vi "laser-shutter-control-subvi.vi"(7 "Camera Shutter":bool, 8 "error in":errorcluster, 9 "VISA resource name out":refnum<visa-resource-name>, 10 "Wheel Speed":u8, 11 "Laser Shutter":T1) -> (0 "error out":errorcluster, 1 "Status":bool, 3 "Current Filterwheel":string)   [LabVIEW 2014]
uses:
  ctts/laser shutters.ctl
  Global Shutter Variables - SubVI.vi
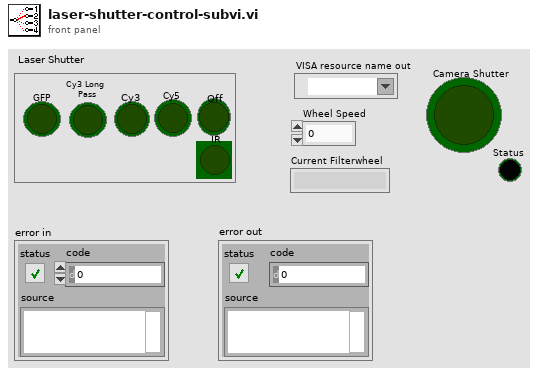
[diagram p1: front panel]
types:
  T1 = typedef "laser shutters.ctl" = enum32{"No Selection", "GFP", "Cy3 Long \nPass", "Cy3", "Cy5", "Off", "IR"}
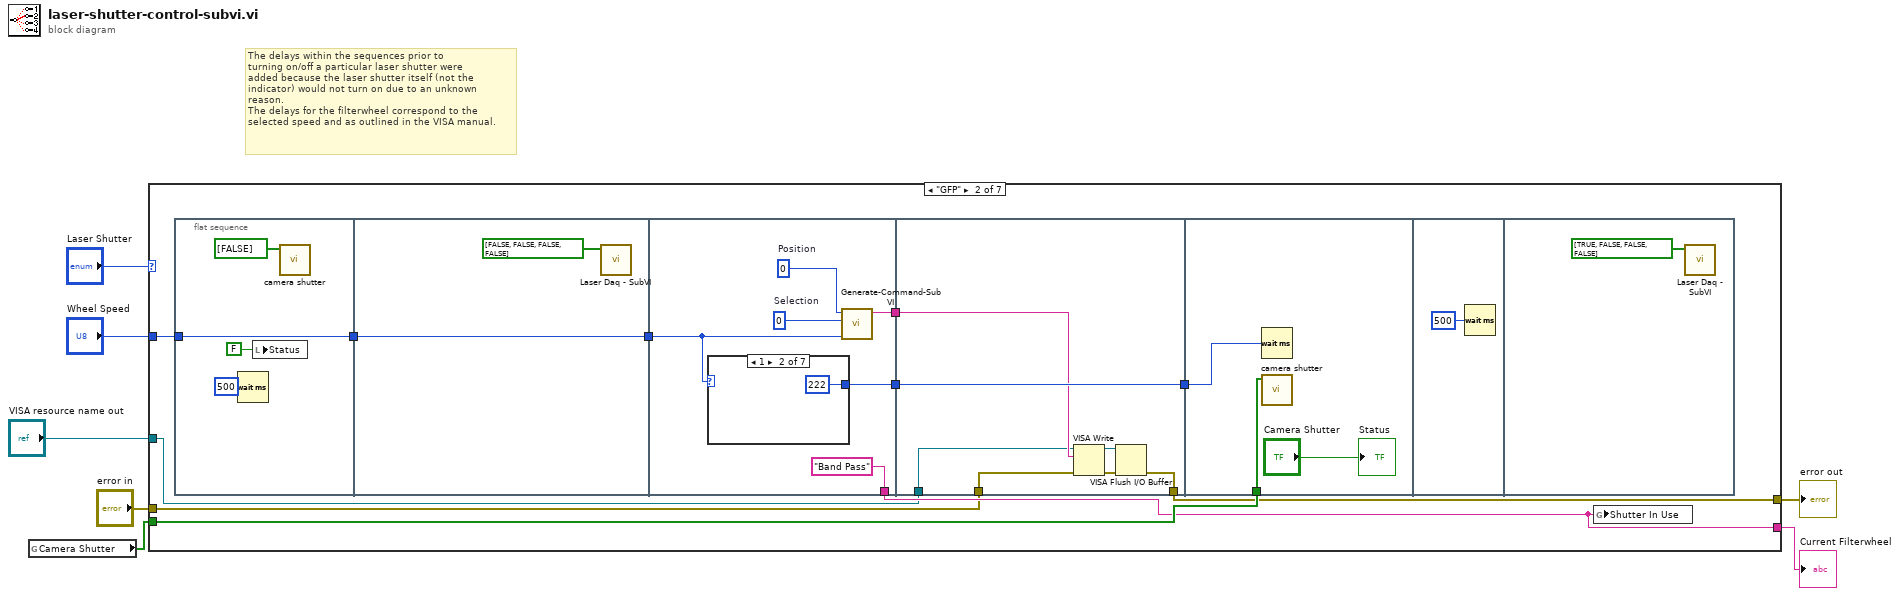
[diagram p0: block diagram]
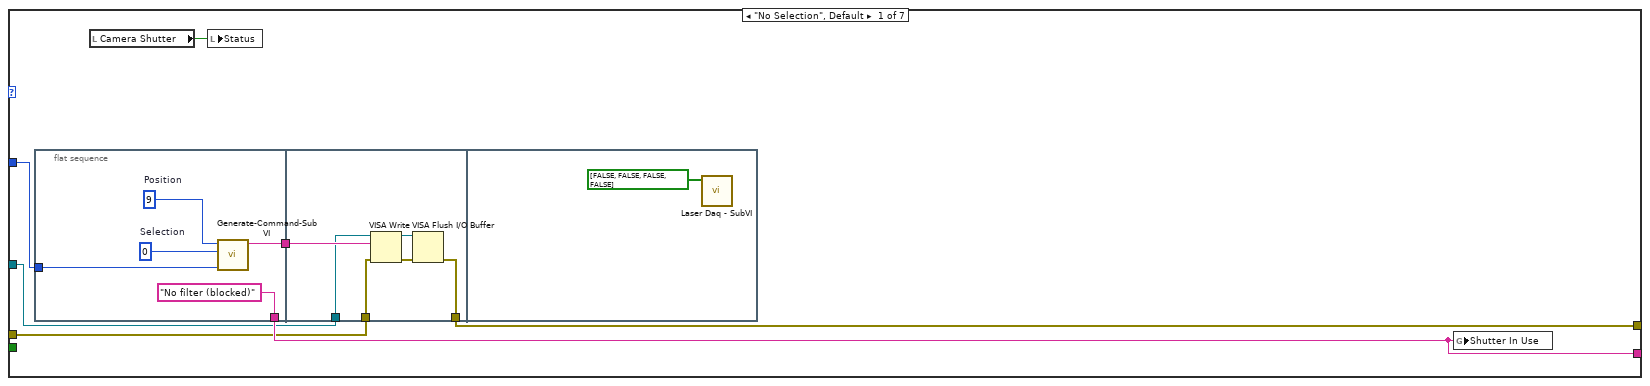
[diagram p2: hidden frame]
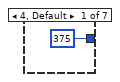
[diagram p3: hidden frame]
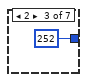
[diagram p4: hidden frame]
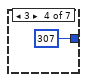
[diagram p5: hidden frame]
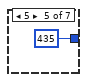
[diagram p6: hidden frame]
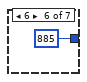
[diagram p7: hidden frame]
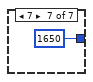
[diagram p8: hidden frame]
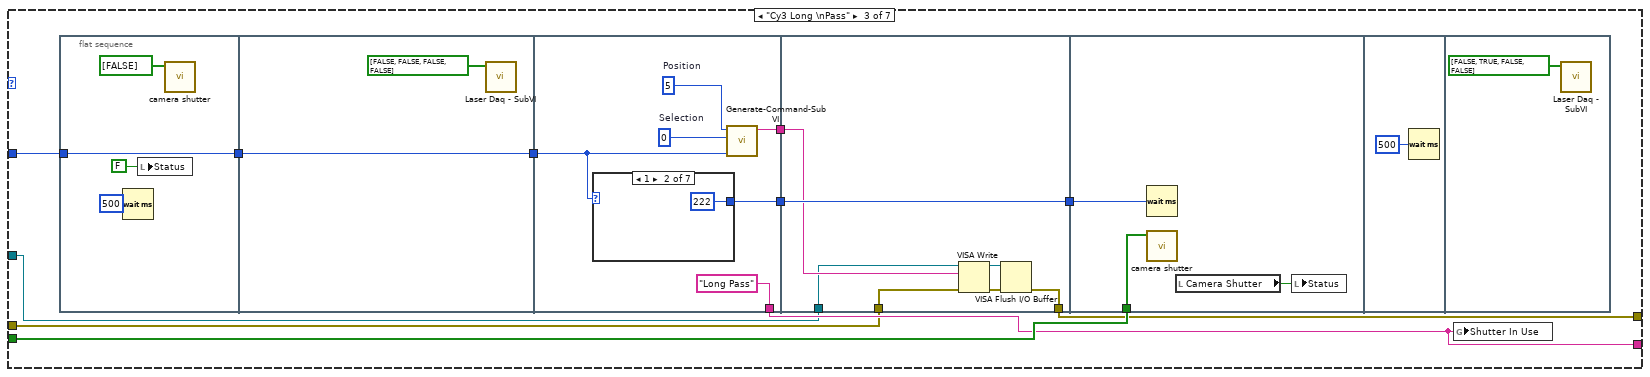
[diagram p9: hidden frame]
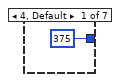
[diagram p10: hidden frame]
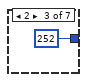
[diagram p11: hidden frame]
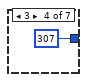
[diagram p12: hidden frame]
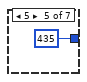
[diagram p13: hidden frame]
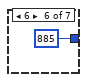
[diagram p14: hidden frame]
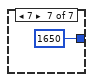
[diagram p15: hidden frame]
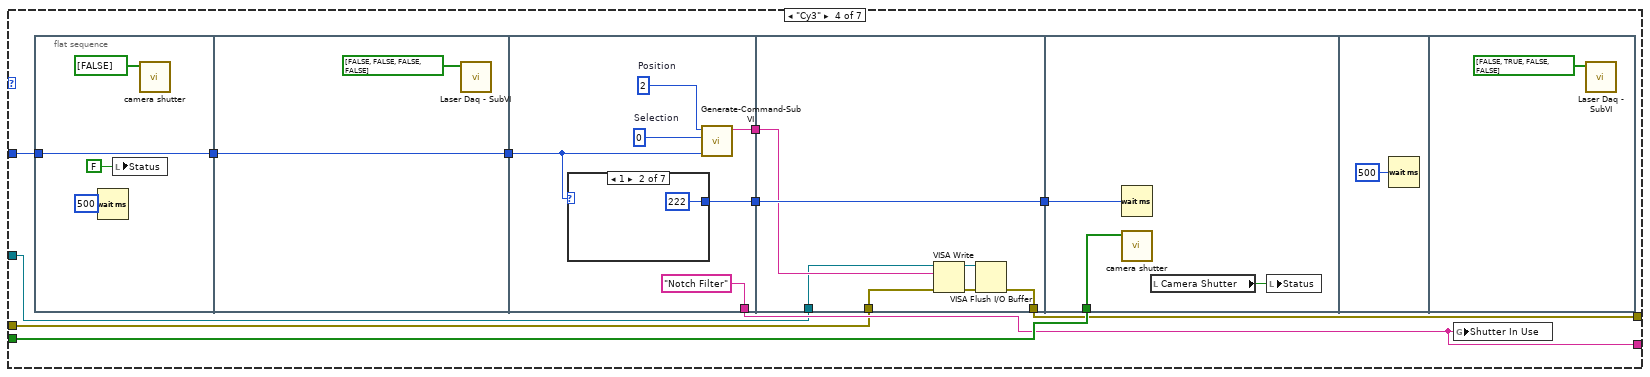
[diagram p16: hidden frame]
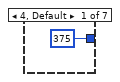
[diagram p17: hidden frame]
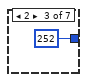
[diagram p18: hidden frame]
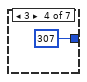
[diagram p19: hidden frame]
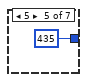
[diagram p20: hidden frame]
diagram:
  # "The delays within the sequences prior to\nturning on/off a particular laser shutter were\nadded because the laser shutter itself (not the\nindicator) would not turn on due to an unknown\nreason. \nThe delays for the filterwheel correspond to the\nselected speed and as outlined in the VISA manual."
  n1 = global read "Global Shutter Variables - SubVI.vi" "Camera Shutter"() -> (w5:bool[])
  n2 = case shown="\"GFP\"" "Laser Shutter" {
    tunnel: "Wheel Speed" -> [w13 w36 w77 w118 w161 w202 w242]
    tunnel: w5 -> [_ w34 w76 w119 w160 w205 _]
    tunnel: "VISA resource name out" -> [w11 w29 w71 w113 w156 w198 w239]
    tunnel: "error in" -> [w10 w28 w70 w112 w154 w197 w238]
    tunnel: [w9 w27 w69 w111 w153 w196 w237] -> w1
    tunnel: [w14 w33 w75 w117 w159 w204 w241] -> w2
    frame "No Selection", Default {
      n3 = flat-sequence {
        tunnel: ["No filter (blocked)"] -> w14
        tunnel: w13 -> [w16]
        tunnel: [w15] -> w12
        tunnel: w12 -> [w23]
        tunnel: w11 -> [w22]
        tunnel: w10 -> [w21]
        tunnel: [w20] -> w9
        frame #0 {
          w17 = 0  # Selection
          w18 = 9  # Position
          n4 = call "Generate-Command-SubVI.vi"("Wheel Speed"=w16, "Wheel Selection"=w17, "Wheel Position"=w18) -> ("type"=w15:string)  [unwired: 8 in]
        }
        frame #1 {
          n5 = VISA Write(VISA resource name=w22, write buffer=w23, error in (no error)=w21) -> (VISA resource name out=w25:refnum<visa-resource-name>, error out=w24:errorcluster)  [unwired: 1 out]
          n6 = VISA Flush I/O Buffer(VISA resource name=w25, error in (no error)=w24) -> (error out=w20:errorcluster)  [unwired: 1 in, 1 out]
        }
        frame #2 {
          n7 = call "Laser Daq - SubVI.vi"("Laser Shutters"=bool[] [FALSE, FALSE, FALSE, FALSE]) -> ()  [unwired: 11 in]
        }
      }
      n8 = local read "Camera Shutter"() -> (w8:bool)
      n9 = local write "Status"(w8) -> ()
      n10 = global write "Global Shutter Variables - SubVI.vi" "Shutter In Use"(w14) -> ()
    }
    frame "GFP" {
      n11 = flat-sequence {
        tunnel: [w38] -> w37
        tunnel: w36 -> [w38]
        tunnel: w37 -> [w42]
        tunnel: [w42] -> w35
        tunnel: w35 -> [w47]
        tunnel: [w46] -> w32
        tunnel: ["Band Pass"] -> w33
        tunnel: [w44] -> w30
        tunnel: w32 -> [w63]
        tunnel: [w63] -> w31
        tunnel: w30 -> [w60]
        tunnel: w29 -> [w59]
        tunnel: w28 -> [w58]
        tunnel: [w57] -> w27
        tunnel: w34 -> [w66]
        tunnel: w31 -> [w64]
        frame #0 {
          n12 = Wait (ms)(milliseconds to wait=500) -> ()  [unwired: 1 out]
          n13 = local write "Status"(FALSE) -> ()
          n14 = call "camera shutter.vi"("Camera Input Switch"=bool[] [FALSE]) -> ()  [unwired: 10 in, 1 out]
        }
        frame #1 {
          n15 = call "Laser Daq - SubVI.vi"("Laser Shutters"=bool[] [FALSE, FALSE, FALSE, FALSE]) -> ()  [unwired: 11 in]
        }
        frame #2 {
          w48 = 0  # Selection
          w49 = 0  # Position
          n16 = case shown="1" w47 {
            tunnel: [375 222 252 307 435 885 1650] -> w46
            frame 4, Default {
            }
            frame 1 {
            }
            frame 2 {
            }
            frame 3 {
            }
            frame 5 {
            }
            frame 6 {
            }
            frame 7 {
            }
          }
          n17 = call "Generate-Command-SubVI.vi"("Wheel Speed"=w47, "Wheel Selection"=w48, "Wheel Position"=w49) -> ("type"=w44:string)  [unwired: 8 in]
        }
        frame #3 {
          n18 = VISA Write(VISA resource name=w59, write buffer=w60, error in (no error)=w58) -> (VISA resource name out=w61:refnum<visa-resource-name>, error out=w62:errorcluster)  [unwired: 1 out]
          n19 = VISA Flush I/O Buffer(VISA resource name=w61, error in (no error)=w62) -> (error out=w57:errorcluster)  [unwired: 1 in, 1 out]
        }
        frame #4 {
          n20 = Wait (ms)(milliseconds to wait=w64) -> ()  [unwired: 1 out]
          n21 = call "camera shutter.vi"("Camera Input Switch"=w66) -> ()  [unwired: 10 in, 1 out]
          "Status" <- "Camera Shutter"
        }
        frame #5 {
          n22 = Wait (ms)(milliseconds to wait=u32 500) -> ()  [unwired: 1 out]
        }
        frame #6 {
          n23 = call "Laser Daq - SubVI.vi"("Laser Shutters"=bool[] [TRUE, FALSE, FALSE, FALSE]) -> ()  [unwired: 11 in]
        }
      }
      n24 = global write "Global Shutter Variables - SubVI.vi" "Shutter In Use"(w33) -> ()
    }
    frame "Cy3 Long \nPass" {
      n25 = flat-sequence {
        tunnel: [w80] -> w79
        tunnel: w77 -> [w80]
        tunnel: w79 -> [w84]
        tunnel: [w84] -> w78
        tunnel: w78 -> [w89]
        tunnel: [w88] -> w74
        tunnel: ["Long Pass"] -> w75
        tunnel: [w86] -> w72
        tunnel: w74 -> [w105]
        tunnel: [w105] -> w73
        tunnel: w72 -> [w102]
        tunnel: w71 -> [w101]
        tunnel: w70 -> [w100]
        tunnel: [w99] -> w69
        tunnel: w76 -> [w108]
        tunnel: w73 -> [w106]
        frame #0 {
          n26 = Wait (ms)(milliseconds to wait=500) -> ()  [unwired: 1 out]
          n27 = local write "Status"(FALSE) -> ()
          n28 = call "camera shutter.vi"("Camera Input Switch"=bool[] [FALSE]) -> ()  [unwired: 10 in, 1 out]
        }
        frame #1 {
          n29 = call "Laser Daq - SubVI.vi"("Laser Shutters"=bool[] [FALSE, FALSE, FALSE, FALSE]) -> ()  [unwired: 11 in]
        }
        frame #2 {
          w90 = 0  # Selection
          w91 = 5  # Position
          n30 = case shown="1" w89 {
            tunnel: [375 222 252 307 435 885 1650] -> w88
            frame 4, Default {
            }
            frame 1 {
            }
            frame 2 {
            }
            frame 3 {
            }
            frame 5 {
            }
            frame 6 {
            }
            frame 7 {
            }
          }
          n31 = call "Generate-Command-SubVI.vi"("Wheel Speed"=w89, "Wheel Selection"=w90, "Wheel Position"=w91) -> ("type"=w86:string)  [unwired: 8 in]
        }
        frame #3 {
          n32 = VISA Write(VISA resource name=w101, write buffer=w102, error in (no error)=w100) -> (VISA resource name out=w103:refnum<visa-resource-name>, error out=w104:errorcluster)  [unwired: 1 out]
          n33 = VISA Flush I/O Buffer(VISA resource name=w103, error in (no error)=w104) -> (error out=w99:errorcluster)  [unwired: 1 in, 1 out]
        }
        frame #4 {
          n34 = Wait (ms)(milliseconds to wait=w106) -> ()  [unwired: 1 out]
          n35 = call "camera shutter.vi"("Camera Input Switch"=w108) -> ()  [unwired: 10 in, 1 out]
          n36 = local read "Camera Shutter"() -> (w107:bool)
          n37 = local write "Status"(w107) -> ()
        }
        frame #5 {
          n38 = Wait (ms)(milliseconds to wait=u32 500) -> ()  [unwired: 1 out]
        }
        frame #6 {
          n39 = call "Laser Daq - SubVI.vi"("Laser Shutters"=bool[] [FALSE, TRUE, FALSE, FALSE]) -> ()  [unwired: 11 in]
        }
      }
      n40 = global write "Global Shutter Variables - SubVI.vi" "Shutter In Use"(w75) -> ()
    }
    frame "Cy3" {
      n41 = flat-sequence {
        tunnel: [w122] -> w121
        tunnel: w118 -> [w122]
        tunnel: w121 -> [w126]
        tunnel: [w126] -> w120
        tunnel: w120 -> [w131]
        tunnel: [w130] -> w116
        tunnel: ["Notch Filter"] -> w117
        tunnel: [w128] -> w114
        tunnel: w116 -> [w147]
        tunnel: [w147] -> w115
        tunnel: w114 -> [w145]
        tunnel: w113 -> [w144]
        tunnel: w112 -> [w143]
        tunnel: [w141] -> w111
        tunnel: w119 -> [w150]
        tunnel: w115 -> [w148]
        frame #0 {
          n42 = Wait (ms)(milliseconds to wait=500) -> ()  [unwired: 1 out]
          n43 = local write "Status"(FALSE) -> ()
          n44 = call "camera shutter.vi"("Camera Input Switch"=bool[] [FALSE]) -> ()  [unwired: 10 in, 1 out]
        }
        frame #1 {
          n45 = call "Laser Daq - SubVI.vi"("Laser Shutters"=bool[] [FALSE, FALSE, FALSE, FALSE]) -> ()  [unwired: 11 in]
        }
        frame #2 {
          w132 = 0  # Selection
          w133 = 2  # Position
          n46 = case shown="1" w131 {
            tunnel: [375 222 252 307 435 885 1650] -> w130
            frame 4, Default {
            }
            frame 1 {
            }
            frame 2 {
            }
            frame 3 {
            }
            frame 5 {
            }
            frame 6 {
            }
            frame 7 {
            }
          }
          n47 = call "Generate-Command-SubVI.vi"("Wheel Speed"=w131, "Wheel Selection"=w132, "Wheel Position"=w133) -> ("type"=w128:string)  [unwired: 8 in]
        }
        frame #3 {
          n48 = VISA Write(VISA resource name=w144, write buffer=w145, error in (no error)=w143) -> (VISA resource name out=w142:refnum<visa-resource-name>, error out=w146:errorcluster)  [unwired: 1 out]
          n49 = VISA Flush I/O Buffer(VISA resource name=w142, error in (no error)=w146) -> (error out=w141:errorcluster)  [unwired: 1 in, 1 out]
        }
        frame #4 {
          n50 = Wait (ms)(milliseconds to wait=w148) -> ()  [unwired: 1 out]
          n51 = call "camera shutter.vi"("Camera Input Switch"=w150) -> ()  [unwired: 10 in, 1 out]
          n52 = local read "Camera Shutter"() -> (w149:bool)
          n53 = local write "Status"(w149) -> ()
        }
        frame #5 {
          n54 = Wait (ms)(milliseconds to wait=u32 500) -> ()  [unwired: 1 out]
        }
        frame #6 {
          n55 = call "Laser Daq - SubVI.vi"("Laser Shutters"=bool[] [FALSE, TRUE, FALSE, FALSE]) -> ()  [unwired: 11 in]
        }
      }
      n56 = global write "Global Shutter Variables - SubVI.vi" "Shutter In Use"(w117) -> ()
    }
    frame "Cy5" {
      n57 = flat-sequence {
        tunnel: [w164] -> w163
        tunnel: w161 -> [w164]
        tunnel: w163 -> [w168]
        tunnel: [w168] -> w162
        tunnel: w162 -> [w173]
        tunnel: [w172] -> w158
        tunnel: ["Notch Filter"] -> w159
        tunnel: [w170] -> w155
        tunnel: w158 -> [w189]
        tunnel: [w189] -> w157
        tunnel: w156 -> [w187]
        tunnel: w155 -> [w186]
        tunnel: w154 -> [w185]
        tunnel: [w184] -> w153
        tunnel: w160 -> [w192]
        tunnel: w157 -> [w190]
        frame #0 {
          n58 = Wait (ms)(milliseconds to wait=500) -> ()  [unwired: 1 out]
          n59 = local write "Status"(FALSE) -> ()
          n60 = call "camera shutter.vi"("Camera Input Switch"=bool[] [FALSE]) -> ()  [unwired: 10 in, 1 out]
        }
        frame #1 {
          n61 = call "Laser Daq - SubVI.vi"("Laser Shutters"=bool[] [FALSE, FALSE, FALSE, FALSE]) -> ()  [unwired: 11 in]
        }
        frame #2 {
          w174 = 0  # Selection
          w175 = 7  # Position
          n62 = case shown="1" w173 {
            tunnel: [375 222 252 307 435 885 1650] -> w172
            frame 4, Default {
            }
            frame 1 {
            }
            frame 2 {
            }
            frame 3 {
            }
            frame 5 {
            }
            frame 6 {
            }
            frame 7 {
            }
          }
          n63 = call "Generate-Command-SubVI.vi"("Wheel Speed"=w173, "Wheel Selection"=w174, "Wheel Position"=w175) -> ("type"=w170:string)  [unwired: 8 in]
        }
        frame #3 {
          n64 = VISA Write(VISA resource name=w187, write buffer=w186, error in (no error)=w185) -> (VISA resource name out=w183:refnum<visa-resource-name>, error out=w188:errorcluster)  [unwired: 1 out]
          n65 = VISA Flush I/O Buffer(VISA resource name=w183, error in (no error)=w188) -> (error out=w184:errorcluster)  [unwired: 1 in, 1 out]
        }
        frame #4 {
          n66 = Wait (ms)(milliseconds to wait=w190) -> ()  [unwired: 1 out]
          n67 = call "camera shutter.vi"("Camera Input Switch"=w192) -> ()  [unwired: 10 in, 1 out]
          n68 = local read "Camera Shutter"() -> (w191:bool)
          n69 = local write "Status"(w191) -> ()
        }
        frame #5 {
          n70 = Wait (ms)(milliseconds to wait=u32 500) -> ()  [unwired: 1 out]
        }
        frame #6 {
          n71 = call "Laser Daq - SubVI.vi"("Laser Shutters"=bool[] [FALSE, FALSE, TRUE, FALSE]) -> ()  [unwired: 11 in]
        }
      }
      n72 = global write "Global Shutter Variables - SubVI.vi" "Shutter In Use"(w159) -> ()
    }
    frame "IR" {
      n73 = flat-sequence {
        tunnel: [w206] -> w203
        tunnel: w202 -> [w206]
        tunnel: w203 -> [w210]
        tunnel: [w210] -> w201
        tunnel: ["No filter (blocked)"] -> w204
        tunnel: w201 -> [w212]
        tunnel: [w216] -> w200
        tunnel: [w215] -> w195
        tunnel: w200 -> [w231]
        tunnel: [w231] -> w199
        tunnel: w198 -> [w229]
        tunnel: w197 -> [w228]
        tunnel: [w226] -> w196
        tunnel: w195 -> [w225]
        tunnel: w205 -> [w234]
        tunnel: w199 -> [w232]
        frame #0 {
          n74 = Wait (ms)(milliseconds to wait=500) -> ()  [unwired: 1 out]
          n75 = local write "Status"(FALSE) -> ()
          n76 = call "camera shutter.vi"("Camera Input Switch"=bool[] [FALSE]) -> ()  [unwired: 10 in, 1 out]
        }
        frame #1 {
          n77 = call "Laser Daq - SubVI.vi"("Laser Shutters"=bool[] [FALSE, FALSE, FALSE, FALSE]) -> ()  [unwired: 11 in]
        }
        frame #2 {
          w213 = 0  # Selection
          w214 = 9  # Position
          n78 = case shown="1" w212 {
            tunnel: [375 222 252 307 435 885 1650] -> w216
            frame 4, Default {
            }
            frame 1 {
            }
            frame 2 {
            }
            frame 3 {
            }
            frame 5 {
            }
            frame 6 {
            }
            frame 7 {
            }
          }
          n79 = call "Generate-Command-SubVI.vi"("Wheel Speed"=w212, "Wheel Selection"=w213, "Wheel Position"=w214) -> ("type"=w215:string)  [unwired: 8 in]
        }
        frame #3 {
          n80 = VISA Write(VISA resource name=w229, write buffer=w225, error in (no error)=w228) -> (VISA resource name out=w230:refnum<visa-resource-name>, error out=w227:errorcluster)  [unwired: 1 out]
          n81 = VISA Flush I/O Buffer(VISA resource name=w230, error in (no error)=w227) -> (error out=w226:errorcluster)  [unwired: 1 in, 1 out]
        }
        frame #4 {
          n82 = Wait (ms)(milliseconds to wait=w232) -> ()  [unwired: 1 out]
          n83 = call "camera shutter.vi"("Camera Input Switch"=w234) -> ()  [unwired: 10 in, 1 out]
          n84 = local read "Camera Shutter"() -> (w233:bool)
          n85 = local write "Status"(w233) -> ()
        }
        frame #5 {
          n86 = Wait (ms)(milliseconds to wait=u32 500) -> ()  [unwired: 1 out]
        }
        frame #6 {
          n87 = call "Laser Daq - SubVI.vi"("Laser Shutters"=bool[] [FALSE, FALSE, FALSE, TRUE]) -> ()  [unwired: 11 in]
        }
      }
    }
    frame "Off" {
      n88 = flat-sequence {
        tunnel: w242 -> [w245]
        tunnel: ["No filter (blocked)"] -> w241
        tunnel: [w243] -> w240
        tunnel: w240 -> [w251]
        tunnel: w239 -> [w250]
        tunnel: w238 -> [w249]
        tunnel: [w248] -> w237
        frame #0 {
          w246 = 0  # Selection
          w247 = 9  # Position
          n89 = call "Generate-Command-SubVI.vi"("Wheel Speed"=w245, "Wheel Selection"=w246, "Wheel Position"=w247) -> ("type"=w243:string)  [unwired: 8 in]
        }
        frame #1 {
          n90 = VISA Write(VISA resource name=w250, write buffer=w251, error in (no error)=w249) -> (VISA resource name out=w253:refnum<visa-resource-name>, error out=w252:errorcluster)  [unwired: 1 out]
          n91 = VISA Flush I/O Buffer(VISA resource name=w253, error in (no error)=w252) -> (error out=w248:errorcluster)  [unwired: 1 in, 1 out]
        }
        frame #2 {
          w255 = bool[] [FALSE]
          w254 = FALSE
          n92 = call "camera shutter.vi"("Camera Input Switch"=w255) -> ()  [unwired: 10 in, 1 out]
          n93 = global write "Global Shutter Variables - SubVI.vi" "Camera Shutter"(w255) -> ()
          n94 = local write "Status"(w254) -> ()
          n95 = local write "Camera Shutter"(w254) -> ()
        }
        frame #3 {
          n96 = call "Laser Daq - SubVI.vi"("Laser Shutters"=bool[] [FALSE, FALSE, FALSE, FALSE]) -> ()  [unwired: 11 in]
        }
      }
      n97 = global write "Global Shutter Variables - SubVI.vi" "Shutter In Use"(w241) -> ()
    }
  }
  "Current Filterwheel" <- w2
  "error out" <- w1
